vi "Get Status Color.vi"(1 "Monkey Status":T1) -> (0 "Color":u32(colorbox)=16777225)   [LabVIEW 2020, in "Tamer.lvlib" / "Tamer.lvclass"]
uses:
  Tamer.lvclass
  Run Utilities/TypeDefs/Monkey Status.ctl
  Run Utilities/Run Utilities.lvlib
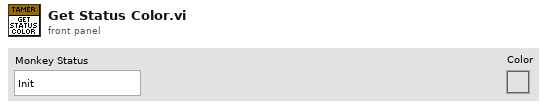
[diagram p1: front panel]
types:
  T1 = typedef "TALOS.lvlib/Run Utilities.lvlib/Monkey Status.ctl" = enum16{"Init", "Paused", "Ongoing", "Stopped", "Finished (no errors)", "Finished (with errors)"}
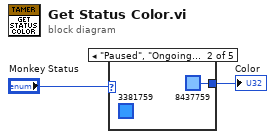
[diagram p0: block diagram]
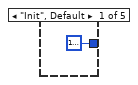
[diagram p2: hidden frame]
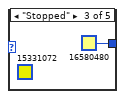
[diagram p3: hidden frame]
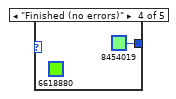
[diagram p4: hidden frame]
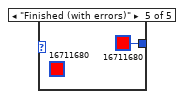
[diagram p5: hidden frame]
diagram:
  n1 = case shown="\"Paused\", \"Ongoing\"" "Monkey Status" {
    tunnel: [u32 16777225 ("Color") u32 8437759 ("Color") u32 16580480 ("Color") u32 8454019 ("Color") u32 16711680 ("Color")] -> w2
    frame "Init", Default {
    }
    frame "Paused", "Ongoing" {
      (unwired) u32 3381759 ("Color")
    }
    frame "Stopped" {
      (unwired) u32 15331072 ("Color")
    }
    frame "Finished (no errors)" {
      (unwired) u32 6618880 ("Color")
    }
    frame "Finished (with errors)" {
      (unwired) u32 16711680 ("Color")
    }
  }
  "Color" <- w2
